vi "428_READER_HW.vi"(8 "error in (no error)":errorcluster, 9 "Command 2":string, 10 "Command 1":string, 11 "VISA resource name":refnum<visa-resource-name>) -> (0 "error out":errorcluster, 1 "Power":string, 2 "Wavelength":string="0000.0000\r\n", 3 "VISA resource name out":refnum<visa-resource-name>)   [LabVIEW 2016]
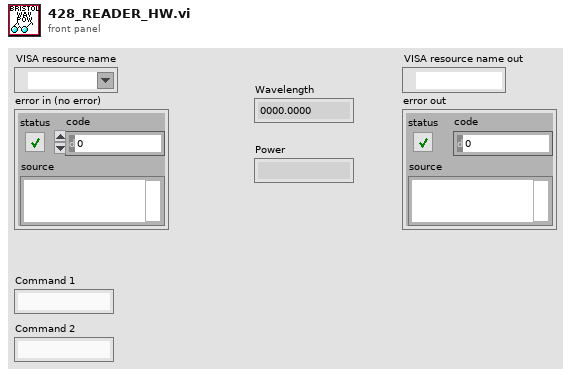
[diagram p1: front panel]
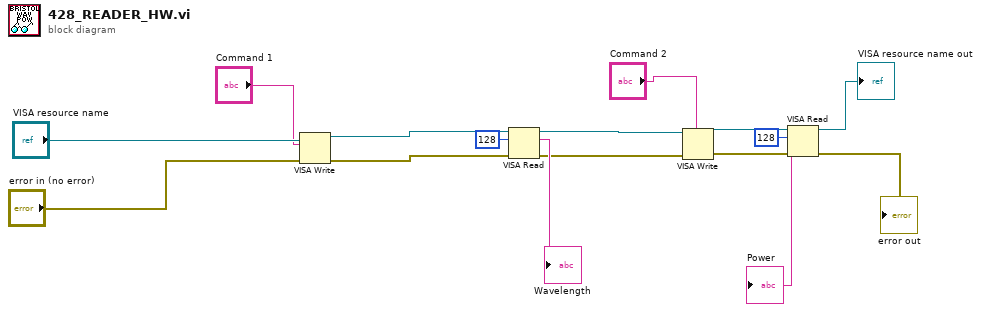
[diagram p0: block diagram]
diagram:
  n1 = VISA Write(VISA resource name="VISA resource name", write buffer="Command 1", error in (no error)="error in (no error)") -> (VISA resource name out=w16:refnum<visa-resource-name>, error out=w15:errorcluster)  [unwired: 1 out]
  n2 = VISA Read(VISA resource name=w16, byte count=u32 128, error in (no error)=w15) -> (VISA resource name out=w12:refnum<visa-resource-name>, read buffer=→"Wavelength":string, error out=w11:errorcluster)  [unwired: 1 out]
  n3 = VISA Write(VISA resource name=w12, write buffer="Command 2", error in (no error)=w11) -> (VISA resource name out=w10:refnum<visa-resource-name>, error out=w9:errorcluster)  [unwired: 1 out]
  n4 = VISA Read(VISA resource name=w10, byte count=u32 128, error in (no error)=w9) -> (VISA resource name out=→"VISA resource name out":refnum<visa-resource-name>, read buffer=→"Power":string, error out=→"error out":errorcluster)  [unwired: 1 out]
